vi "svx_DAQ_SetTimingCaptions.vi"(0 "Timing Mode (new)":T1 caption="Mode", 5 "Timing Mode (old)":T1 caption="Mode", 9 "Reference Cluster":T2, 11 "error in (no error)":errorcluster) -> (4 "Timing Control 1":dbl, 6 "Timing Control 2":dbl, 8 "Timing Control 3":i32, 10 "Reference Cluster Out":T2, 15 "error out":errorcluster)   [LabVIEW 2017, in "SVX NI-DAQmx AI Configuration XControl.xctl"]
uses:
  <vilib>/addons/Sound and Vibration/svt_DAQmx/Configuration XControl/SVX NI-DAQmx AI Configuration XControl.xctl
  <vilib>/addons/Sound and Vibration/svt_DAQmx/Configuration XControl/Controls/svx_DAQ_ControlRefs.ctl
  <vilib>/addons/Sound and Vibration/svt_DAQmx/Configuration XControl/Controls/svx_DAQ_ChannelInfo.ctl
  <vilib>/addons/Sound and Vibration/svt_DAQmx/Configuration XControl/Controls/svx_DAQ_ChannelType.ctl
  <vilib>/addons/Sound and Vibration/svt_DAQmx/Configuration XControl/Controls/svx_DAQ_Coupling.ctl
  <vilib>/addons/Sound and Vibration/svt_DAQmx/Configuration XControl/Controls/svx_DAQ_Excitation.ctl
  <vilib>/addons/Sound and Vibration/svt_DAQmx/Configuration XControl/Controls/svx_DAQ_TimingType.ctl
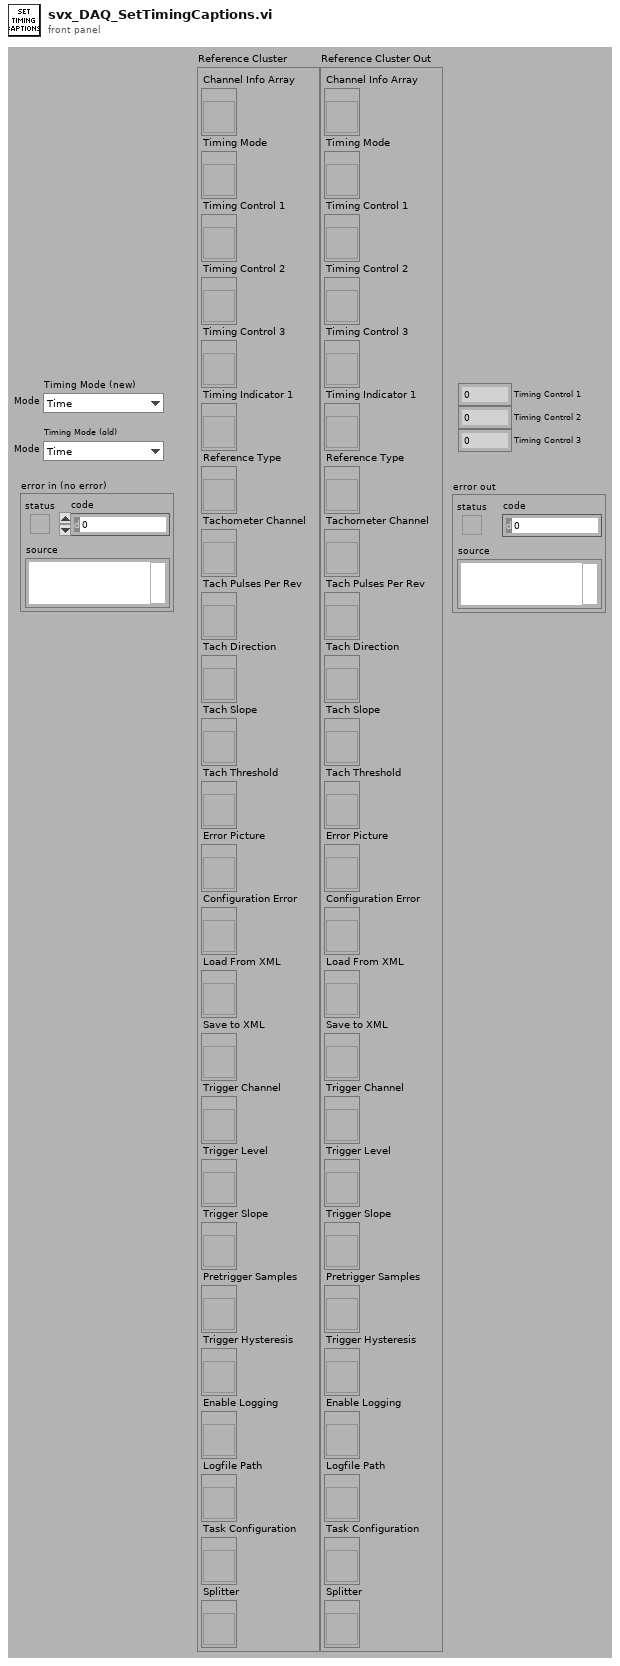
[diagram p1: front panel]
types:
  T1 = typedef "SVX NI-DAQmx AI Configuration XControl.xctl/svx_DAQ_TimingType.ctl" = enum16{"Time", "Frequency", "Order"}
  T2 = typedef "SVX NI-DAQmx AI Configuration XControl.xctl/svx_DAQ_ControlRefs.ctl" = cluster{"Channel Info Array":refnum<vi>, "Timing Mode":refnum<vi>, "Timing Control 1":refnum<vi>, "Timing Control 2":refnum<vi>, "Timing Control 3":refnum<vi>, "Timing Indicator 1":refnum<vi>, "Reference Type":refnum<vi>, "Tachometer Channel":refnum<vi>, "Tach Pulses Per Rev":refnum<vi>, "Tach Direction":refnum<vi>, "Tach Slope":refnum<vi>, "Tach Threshold":refnum<vi>, "Error Picture":refnum<vi>, "Configuration Error":refnum<vi>, "Load From XML":refnum<vi>, "Save to XML":refnum<vi>, "Trigger Channel":refnum<vi>, "Trigger Level":refnum<vi>, "Trigger Slope":refnum<vi>, "Pretrigger Samples":refnum<vi>, "Trigger Hysteresis":refnum<vi>, "Enable Logging":refnum<vi>, "Logfile Path":refnum<vi>, "Task Configuration":refnum<vi>, "Splitter":refnum<vi>}
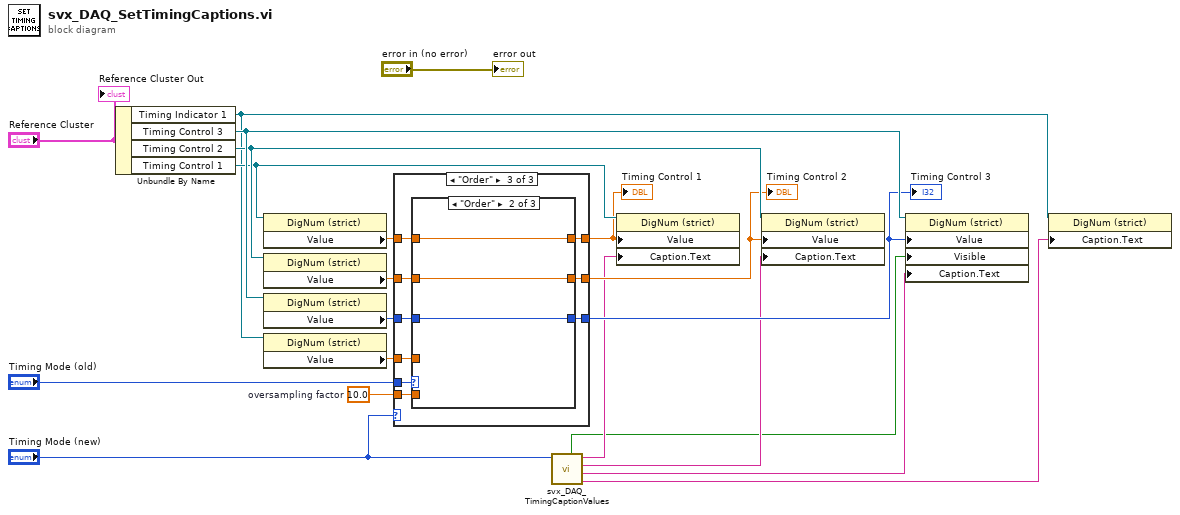
[diagram p0: block diagram]
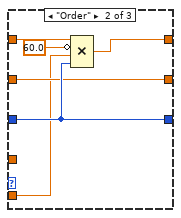
[diagram p3: hidden frame]
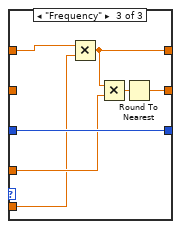
[diagram p4: hidden frame]
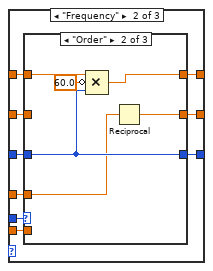
[diagram p5: hidden frame]
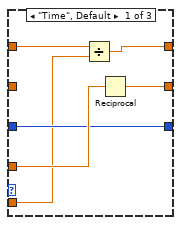
[diagram p6: hidden frame]
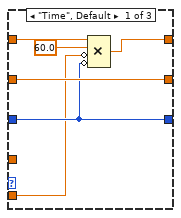
[diagram p8: hidden frame]
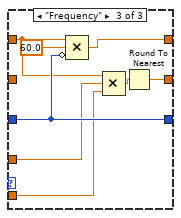
[diagram p9: hidden frame]
diagram:
  w9 = 10.0  # oversampling factor
  n1 = Unbundle By Name("Reference Cluster") -> ("Timing Indicator 1"=w17:refnum<vi>, "Timing Control 3"=w20:refnum<vi>, "Timing Control 2"=w19:refnum<vi>, "Timing Control 1"=w18:refnum<vi>)
  n2 = property class="DigNum (strict)"(reference=w18) -> ("Value"=w16:dbl)  [unwired: 1 in, 2 out]
  n3 = property class="DigNum (strict)"(reference=w19) -> ("Value"=w14:dbl)  [unwired: 1 in, 2 out]
  n4 = property class="DigNum (strict)"(reference=w20) -> ("Value"=w13:i32)  [unwired: 1 in, 2 out]
  n5 = property class="DigNum (strict)"(reference=w17) -> ("Value"=w12:dbl)  [unwired: 1 in, 2 out]
  n6 = case shown="\"Order\"" "Timing Mode (new)" {
    tunnel: "Timing Mode (old)" -> [w26 w55 w79]
    tunnel: w16 -> [w30 w54 w78]
    tunnel: [w25 w53 w72] -> w15
    tunnel: w14 -> [w29 w52 w77]
    tunnel: w13 -> [w28 w51 w76]
    tunnel: w12 -> [w27 w50 w75]
    tunnel: [w24 w49 w73] -> w11
    tunnel: [w23 w48 w74] -> w10
    tunnel: w9 -> [w22 w47 w71]
    frame "Time", Default {
      n7 = case shown="\"Time\", Default" w26 {
        tunnel: w30 -> [w33 w39 w45]
        tunnel: [w33 w37 w44] -> w25
        tunnel: w29 -> [w32 w35 _]
        tunnel: w28 -> [w31 w36 w46]
        tunnel: w27 -> [_ _ w43]
        tunnel: [w32 w35 w41] -> w24
        tunnel: [w31 w36 w46] -> w23
        tunnel: w22 -> [_ w34 w40]
        frame "Time", Default {
        }
        frame "Order" {
          n8 = Compound Arithmetic op=MULTIPLY(w39, invert 60.0 ("value"), w34, w36) -> (w37:dbl)
        }
        frame "Frequency" {
          n9 = Multiply(x=w45, y=w40) -> (x*y=w44:dbl)
          n10 = Multiply(x=w44, y=w43) -> (x*y=w42:dbl)
          n11 = Round To Nearest(number=w42) -> (nearest integer value=w41:dbl)
        }
      }
    }
    frame "Frequency" {
      n12 = case shown="\"Order\"" w55 {
        tunnel: w54 -> [w59 w67 w70]
        tunnel: [w58 w65 w70] -> w53
        tunnel: w52 -> [_ _ w69]
        tunnel: w51 -> [w57 w64 w68]
        tunnel: w50 -> [w61 w62 _]
        tunnel: [w60 w63 w69] -> w49
        tunnel: [w57 w64 w68] -> w48
        tunnel: w47 -> [w56 _ _]
        frame "Time", Default {
          n13 = Divide(x=w59, y=w56) -> (x/y=w58:dbl)
          n14 = Reciprocal(x=w61) -> (1/x=w60:dbl)
        }
        frame "Order" {
          n15 = Compound Arithmetic op=MULTIPLY(w67, invert 60.0 ("value"), w64) -> (w65:dbl)
          n16 = Reciprocal(x=w62) -> (1/x=w63:dbl)
        }
        frame "Frequency" {
        }
      }
    }
    frame "Order" {
      n17 = case shown="\"Order\"" w79 {
        tunnel: w78 -> [w85 w86 w91]
        tunnel: [w83 w86 w93] -> w72
        tunnel: w77 -> [w82 w87 _]
        tunnel: w76 -> [w81 w88 w95]
        tunnel: w75 -> [_ _ w90]
        tunnel: [w82 w87 w92] -> w73
        tunnel: [w81 w88 w95] -> w74
        tunnel: w71 -> [w80 _ w89]
        frame "Time", Default {
          n18 = Compound Arithmetic op=MULTIPLY(w85, 60.0 ("y"), invert w80, invert w81) -> (w83:dbl)
        }
        frame "Order" {
        }
        frame "Frequency" {
          n19 = Compound Arithmetic op=MULTIPLY(w91, 60.0 ("value"), invert w95) -> (w93:dbl)
          n20 = Compound Arithmetic op=MULTIPLY(w91, w90, w89) -> (w94:dbl)
          n21 = Round To Nearest(number=w94) -> (nearest integer value=w92:dbl)
        }
      }
    }
  }
  "Timing Control 1" <- w15
  "Timing Control 2" <- w11
  "Timing Control 3" <- w10
  n22 = call <vilib>:"svx_DAQ_TimingCaptionValues.vi"("Timing Mode"="Timing Mode (new)") -> ("Timing Indicator 1 Caption"=w2:string, "Timing Control 3 Caption"=w3:string, "Timing Control 2 Caption"=w4:string, "Timing Control 1 Caption"=w5:string, "Timing Control 3 Visible?"=w1:bool)  [unwired: 6 in]
  n23 = property class="DigNum (strict)"(reference=w18, "Value"=w15, "Caption.Text"=w5) -> ()  [unwired: 1 in, 2 out]
  n24 = property class="DigNum (strict)"(reference=w19, "Value"=w11, "Caption.Text"=w4) -> ()  [unwired: 1 in, 2 out]
  n25 = property class="DigNum (strict)"(reference=w20, "Value"=w10, "Visible"=w1, "Caption.Text"=w3) -> ()  [unwired: 1 in, 2 out]
  n26 = property class="DigNum (strict)"(reference=w17, "Caption.Text"=w2) -> ()  [unwired: 1 in, 2 out]
  "error out" <- "error in (no error)"
  "Reference Cluster Out" <- "Reference Cluster"
